vi "GUI Connections.vi"() -> ()   [LabVIEW 2020]
panel:
  out "connections picture":picture
  in  "hide":bool
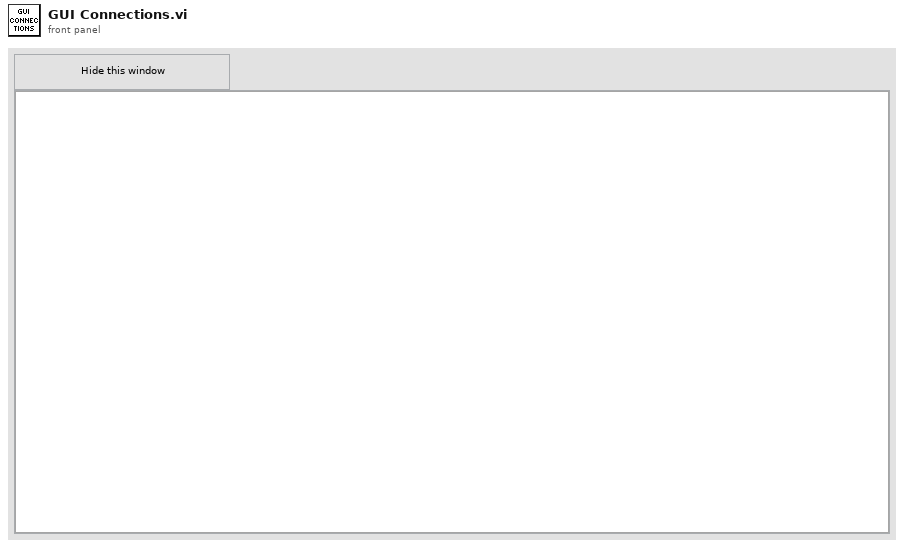
[diagram p1: front panel]
types:
  T1 = typedef "imagedata.ctl" = cluster{"image type":i32, "image depth":i32, "image":u8[], "mask":u8[], "colors":u32[], "Rectangle":cluster{"left":i16, "top":i16, "right":i16, "bottom":i16}}
  T2 = enum32{"Invalid", "Standard", "Closed", "Hidden", "Minimized", "Maximized"}
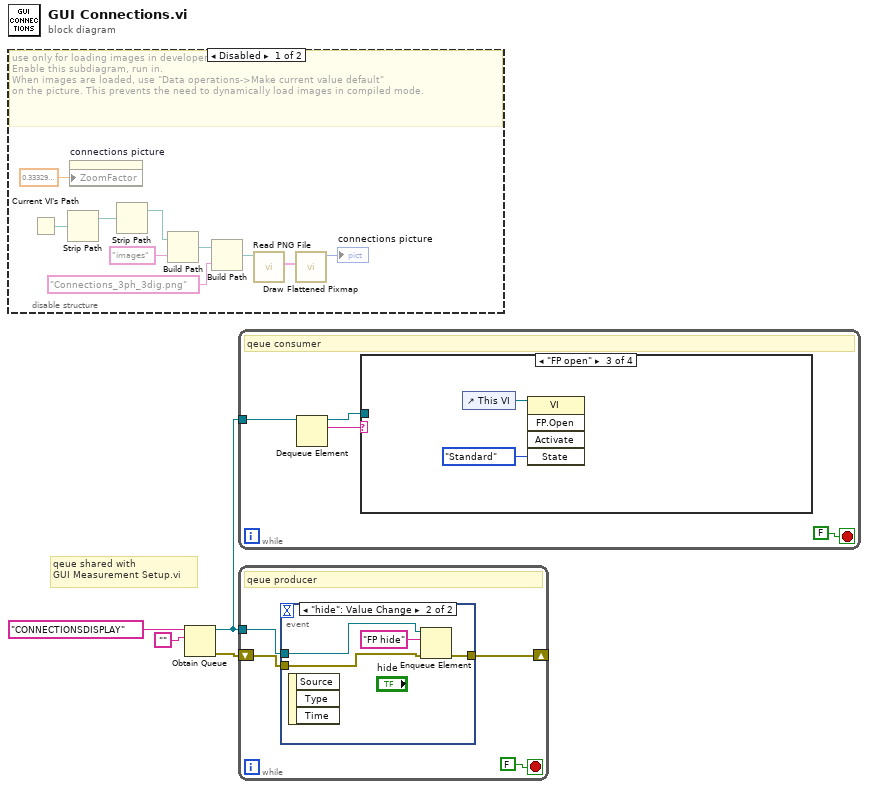
[diagram p0: block diagram]
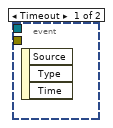
[diagram p2: hidden frame]
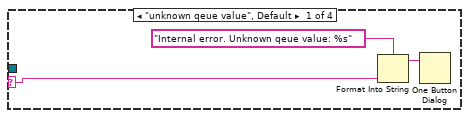
[diagram p3: hidden frame]
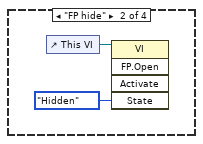
[diagram p4: hidden frame]
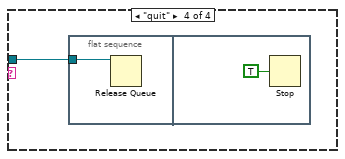
[diagram p5: hidden frame]
diagram:
  # "qeue shared with\nGUI Measurement Setup.vi"
  n1 = disable-structure shown="Disabled" {
    frame Disabled {
      # "use only for loading images in developement mode.\nEnable this subdiagram, run in.\nWhen images are loaded, use \"Data operations->Make current value default\" \non the picture. This prevents the need to dynamically load images in compiled mode."
      n2 = Current VI's Path() -> (path=w14:path)
      n3 = Strip Path(path=w14) -> (stripped path=w13:path)  [unwired: 1 out]
      n4 = property on="connections picture" class="Pict"("ZoomFactor"=sgl 0.3333 ("Zoom Factor")) -> ()  [unwired: 2 in, 2 out]
      n5 = Strip Path(path=w13) -> (stripped path=w12:path)  [unwired: 1 out]
      n6 = Build Path(base path=w12, name or relative path="images") -> (appended path=w7:path)
      n7 = Build Path(base path=w7, name or relative path="Connections_3ph_3dig.png") -> (appended path=w8:path)
      n8 = call <vilib>:"Read PNG File.vi"("path to PNG file"=w8) -> ("image data"=w9:T1)  [unwired: 8 in, 2 out]
      n9 = call <vilib>:"Draw Flattened Pixmap.vi"("image data"=w9) -> ("new picture"=→"connections picture":picture)  [unwired: 8 in]
    }
    frame Enabled {
    }
  }
  n10 = Obtain Queue(name (unnamed)="CONNECTIONSDISPLAY", element data type="" ("data (can be any type)")) -> (queue out=w1:refnum<queue>, error out=w2:errorcluster)  [unwired: 3 in, 1 out]
  n11 = while {
    tunnel: w1 -> [w17]
    stop <- FALSE stop-if-true
    # "qeue consumer"
    n12 = Dequeue Element(queue=w17) -> (queue out=w15:refnum<queue>, element=w16:string)  [unwired: 2 in, 2 out]
    n13 = case shown="\"FP open\"" w16 {
      selector: w16 -> [w19 _ _ _]
      tunnel: w15 -> [_ _ _ w26]
      frame "unknown qeue value", Default {
        n14 = Format Into String(format string="Internal error. Unknown qeue value: %s", w19) -> (resulting string=w21:string)  [unwired: 2 in, 1 out]
        n15 = One Button Dialog(message=w21) -> ()  [unwired: 1 in, 1 out]
      }
      frame "FP hide" {
        n16 = control-ref of="This VI"() -> (w22:refnum<vi>)
        n17 = invoke class="VI" method="FP.Open"(reference=w22, "State"=T2."Hidden") -> ()  [unwired: 3 in, 5 out]
      }
      frame "FP open" {
        n18 = control-ref of="This VI"() -> (w24:refnum<vi>)
        n19 = invoke class="VI" method="FP.Open"(reference=w24, "State"=T2."Standard") -> ()  [unwired: 3 in, 5 out]
      }
      frame "quit" {
        n20 = flat-sequence {
          tunnel: w26 -> [w27]
          frame #0 {
            n21 = Release Queue(queue=w27) -> ()  [unwired: 2 in, 3 out]
          }
          frame #1 {
            n22 = Stop(stop? (T)=TRUE) -> ()
          }
        }
      }
    }
  }
  n23 = while {
    shift-right: [w31] -> _
    shift-left: w2 -> [w32]
    tunnel: w1 -> [w30]
    stop <- FALSE stop-if-true
    # "qeue producer"
    n24 = event shown="[1] \"hide\": Value Change" {
      selector: _ -> [_ _]
      dyn-events: _ -> [_ _]
      timeout: _ -> [_ _]
      tunnel: w32 -> [_ w35]
      tunnel: [_ w34] -> w31
      tunnel: w30 -> [_ w33]
      event Timeout {
        n25 = event-data() -> ()  [unwired: 1 in, 3 out]
      }
      event "hide": Value Change {
        n26 = event-data() -> ()  [unwired: 1 in, 3 out]
        n27 = Enqueue Element(queue=w33, element="FP hide", error in (no error)=w35) -> (error out=w34:errorcluster)  [unwired: 1 in, 2 out]
      }
    }
  }
